vi "getLabelObj.vi"(8 "error in (no error)":errorcluster, 11 "ILabelable in":refnum<class "ILabelable.lvclass">) -> (0 "error out":errorcluster, 2 "label":refnum<class "TextDecoration.lvclass">, 3 "ILabelable out":refnum<class "ILabelable.lvclass">)   [LabVIEW 2023, in "TLC_Scripto.lvlib" / "ILabelable.lvclass"]
uses:
  ILabelable.lvclass
  TextDecoration/TextDecoration.lvclass
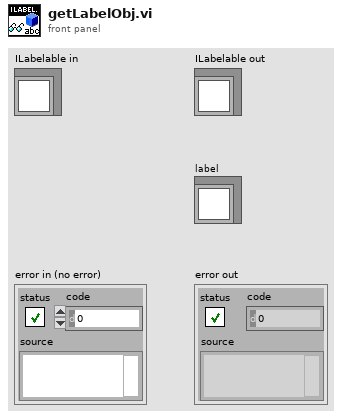
[diagram p1: front panel]
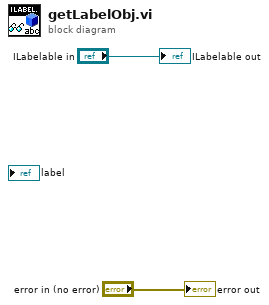
[diagram p0: block diagram]
diagram:
  "error out" <- "error in (no error)"
  "ILabelable out" <- "ILabelable in"
